vi "Main_09A.vi"() -> ()   [LabVIEW 2024]
panel:
  out "Original Array":i32[](array[numeric])
  out "count down":i32
  out "End Array":i32[](array[numeric])
  out "Start Array":i32[](array[numeric])
  in  "Use Puzzle":bool
  out "Answer 6291146824486":u64
  in  "Puzzle":string="231044132293727419353356713211698585172072388022545729466698881739885330345853131193876427493925394014429761602571395381441257752012235131621368478541341764869712703015409959367852508018902266715148819874145969176460451991499162328927998859193886358553338987969221728049824729284712764041946274139389484987606762296286812070559741217532101358588036508666347111484425882317216983675862636276344366502048333862537413316779609175773596178350952698222837837476954334834078386840461362375326798489622437185066581969175658314639521022934457645459938617149663879828547848817873501493208119695668326092176931..."
  in  "Example":string="2333133121414131402"
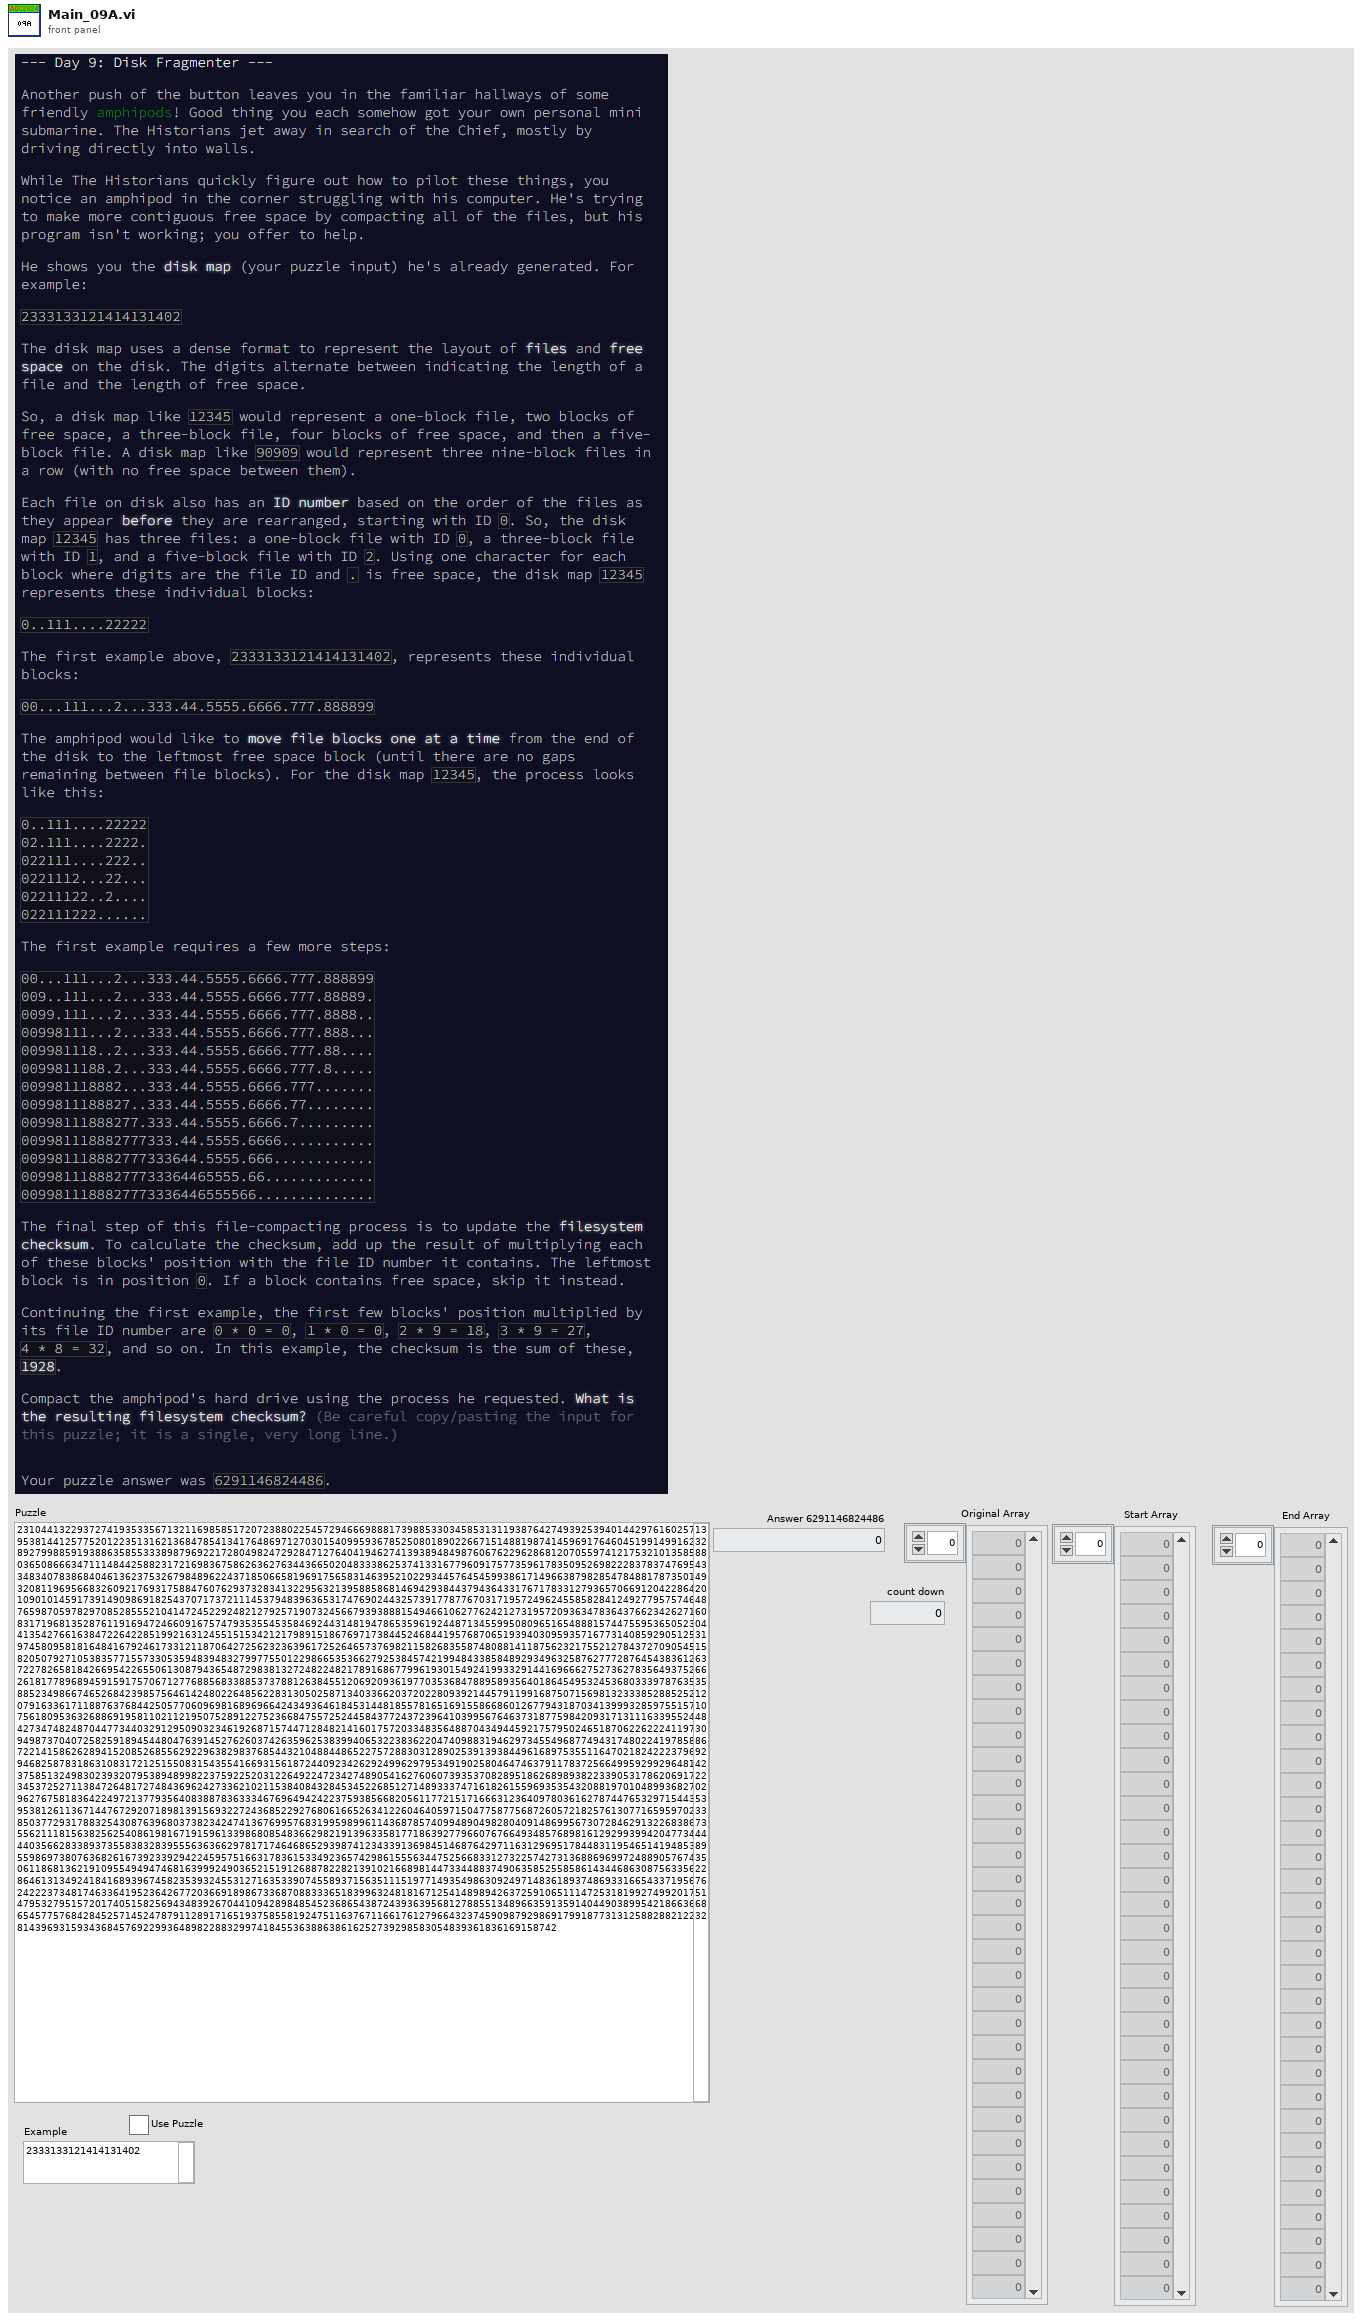
[diagram p1: front panel]
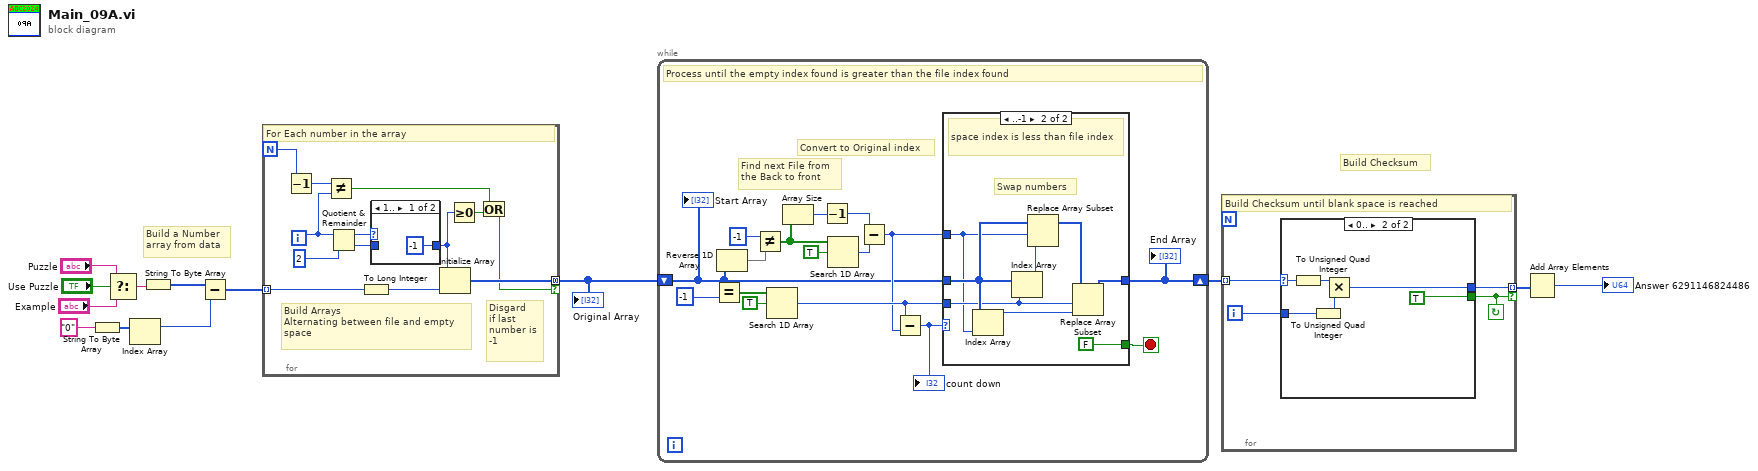
[diagram p0: block diagram]
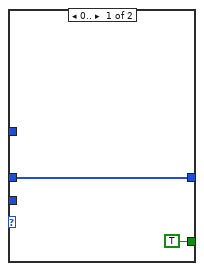
[diagram p3: hidden frame]
diagram:
  # "Build Checksum"
  # "Build a Number\narray from data"
  n1 = String To Byte Array(string="0") -> (unsigned byte array=w7:u8[])
  n2 = Select(t="Puzzle", s="Use Puzzle", f="Example") -> (s? t:f=w9:string)
  n3 = Index Array(array=w7) -> (element=w6:u8)  [unwired: 1 in]
  n4 = String To Byte Array(string=w9) -> (unsigned byte array=w10:u8[])
  n5 = Subtract(x=w10, y=w6) -> (x-y=w5:u8[])
  n6 = for {
    N -> [w20]
    tunnel: w5 -> [w24] mode=indexing
    tunnel: [w22] -> w2 mode=concatenating if=w14
    i -> [w18]
    # "Disgard\nif last\nnumber is\n-1"
    # "Build Arrays\nAlternating between file and empty\nspace"
    # "For Each number in the array"
    n7 = Decrement(x=w20) -> (x-1=w19:i32)
    n8 = Not Equal?(x=w19, y=w18) -> (x != y?=w17:bool)
    n9 = Quotient & Remainder(x=w18, y=2) -> (x-y*floor(x/y)=w25:i32, floor(x/y)=w23:i32)
    n10 = To Long Integer(number=w24) -> (32bit integer=w21:i32)
    n11 = case shown="1.." w25 {
      tunnel: w23 -> [_ w28]
      tunnel: [-1 w28] -> w16
      frame 1.. {
      }
      frame ..0 {
      }
    }
    n12 = Initialize Array(w16, w21) -> (w22:i32[])
    n13 = Greater Or Equal To 0?(x=w16) -> (x >= 0?=w15:bool)
    n14 = Or(x=w17, y=w15) -> (x .or. y?=w14:bool)
  }
  "Original Array" <- w2
  n15 = while {
    shift-right: [w30] -> w4
    shift-left: w2 -> [w29]
    stop <- w31 stop-if-true
    # "Convert to Original index"
    # "Find next File from\nthe Back to front"
    # "Process until the empty index found is greater than the file index found"
    n16 = Equal?(x=w29, y=-1) -> (x = y?=w41:bool[])
    n17 = Reverse 1D Array(array=w29) -> (reversed array=w43:i32[])
    n18 = Not Equal?(x=-1 ("y"), y=w43) -> (x != y?=w40:bool[])
    n19 = Search 1D Array(1D array=w41, element=TRUE) -> (index of element=w34:i32)  [unwired: 1 in]
    n20 = Array Size(array=w40) -> (size(s)=w39:i32)
    n21 = Decrement(x=w39) -> (x-1=w38:i32)
    n22 = Search 1D Array(1D array=w40, element=TRUE) -> (index of element=w35:i32)  [unwired: 1 in]
    n23 = Subtract(x=w38, y=w35) -> (x-y=w33:i32)
    n24 = Subtract(x=w34, y=w33) -> (x-y=w32:i32)
    "count down" <- w32
    n25 = case shown="..-1" w32 {
      tunnel: w29 -> [w46 w54]
      tunnel: w34 -> [_ w53]
      tunnel: [w46 w50] -> w30
      tunnel: w33 -> [_ w48]
      tunnel: [TRUE FALSE] -> w31
      frame 0.. {
      }
      frame ..-1 {
        # "Swap numbers"
        # "space index is less than file index"
        n26 = Index Array(array=w54, index=w48) -> (element=w52:i32)
        n27 = Index Array(array=w54, index=w53) -> (element=w49:i32)
        n28 = Replace Array Subset(array=w54, new element=w49, index=w48) -> (w51:i32[])
        n29 = Replace Array Subset(array=w51, new element=w52, index=w53) -> (w50:i32[])
      }
    }
    "End Array" <- w30
    "Start Array" <- w29
  }
  n30 = for {
    tunnel: w4 -> [w56] mode=indexing
    tunnel: [w58] -> w3 mode=indexing if=w57
    i -> [w55]
    stop <- w57 continue-if-true
    # "Build Checksum until blank space is reached"
    n31 = case shown="0.." w56 {
      selector: w56 -> [_ w64]
      tunnel: [_ w59] -> w58
      tunnel: [_ TRUE] -> w57
      tunnel: w55 -> [_ w61]
      frame ..-1 {
      }
      frame 0.. {
        n32 = To Unsigned Quad Integer(1:w64) -> (0:w62:u64)
        n33 = To Unsigned Quad Integer(1:w61) -> (0:w60:u64)
        n34 = Multiply(x=w62, y=w60) -> (x*y=w59:u64)
      }
    }
  }
  n35 = Add Array Elements(numeric array=w3) -> (sum=→"Answer 6291146824486":u64)
